vi "Address Bond.vi"(6 "Match Offset":cluster{"X":sgl, "Y":sgl}={"X"=-2.0, "Y"=198.0}, 8 "Minimum Match Score":sgl=60.0, 9 "controller in":refnum<k24>, 10 "Template":path, 11 "T/B/L/R":i32) -> (0 "error out":errorcluster, 1 "Number of Matches (Pattern Matching 1)":i32, 3 "Match(es) Found":bool)   [LabVIEW 2011]
uses:
  C:/Users/Admin/Desktop/Gantry Code Transfer/source/Code Transfer/Aerotech.A3200.dll
  Aerotech.A3200.dll
  <vilib>/vision/driver/NI_Vision_Acquisition_Software.lvlib
  <vilib>/vision/NI_Vision_Development_Module.lvlib
panel:
  in  "Scale Factor":sgl=0.000429
  out "y rel move":dbl
  out "x rel move":dbl
  out "y":sgl
  out "x":sgl
  out "Image Out":T1(plugin-control)
  out "Calibrated Matches (Pattern Matching 1)":T2(array[cluster]) {"Bounding Box"."y" format="%.2f"; "Bounding Box"."x" format="%.2f"; "Position"."y" format="%.2f"; "Position"."x" format="%.2f"; "Score" format="%.2f"; "Scale" format="%.2f"; "Angle" format="%.2f"}
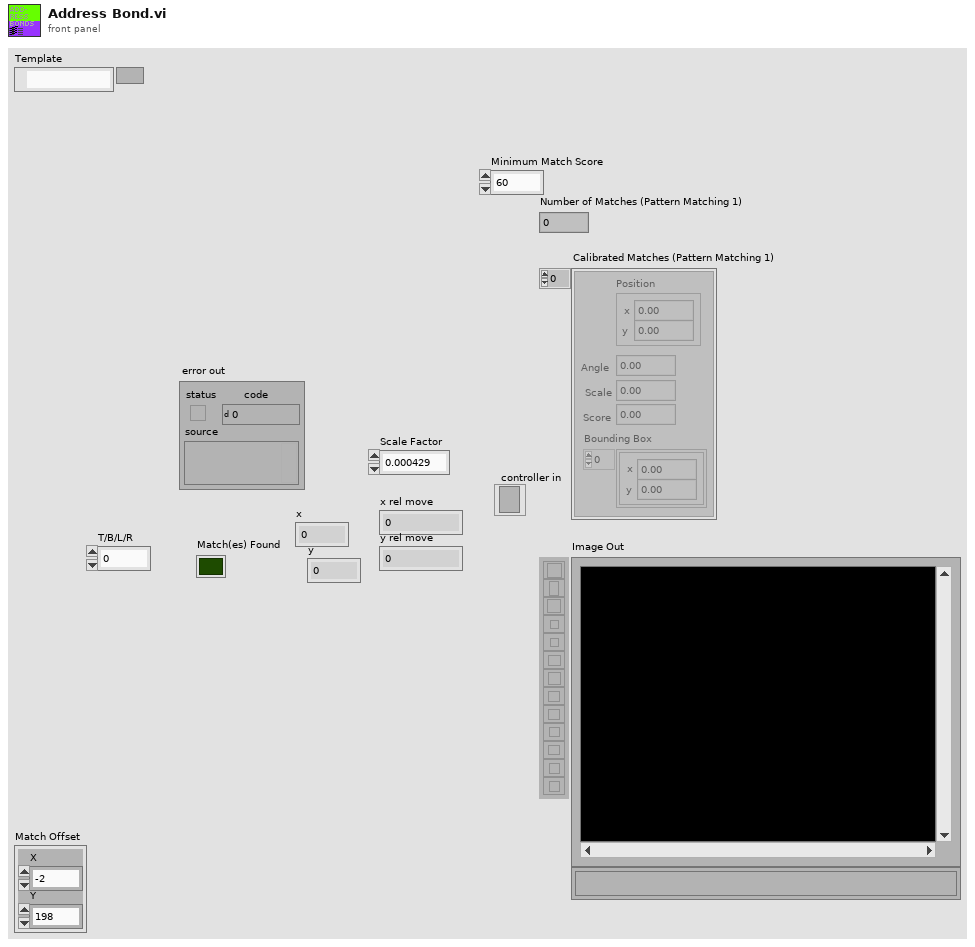
[diagram p1: front panel]
types:
  T1 = typedef "IMAQ Image.ctl" = refnum<image>
  T2 = cluster{"Position":cluster{"x":sgl, "y":sgl}, "Angle":sgl, "Scale":sgl, "Score":sgl, "Bounding Box":cluster{"x":sgl, "y":sgl}[]}[]
  T3 = cluster{"Global Rectangle":i32[], "Contours":cluster{"ID":enum32{"External", "Internal"}, "Type":u32, "Coordinates":i32[]}[]}
  T4 = typedef "IMAQdx.ctl" = refnum<k21>
  T5 = cluster{"Match Mode":u16, "Subpixel Accuracy":bool, "Rotation Angle Ranges (degrees)":cluster{sgl, sgl}[]}
  T6 = cluster{"Global Rectangle":i32[], "Number of Matches Requested":i32, "Minimum Match Score":sgl}
  T7 = cluster{"Position":cluster{"x":sgl, "y":sgl}, "Angle":sgl, "Scale":sgl, "Score":sgl, "Bounding Box":cluster{"x":sgl, "y":sgl}[]}
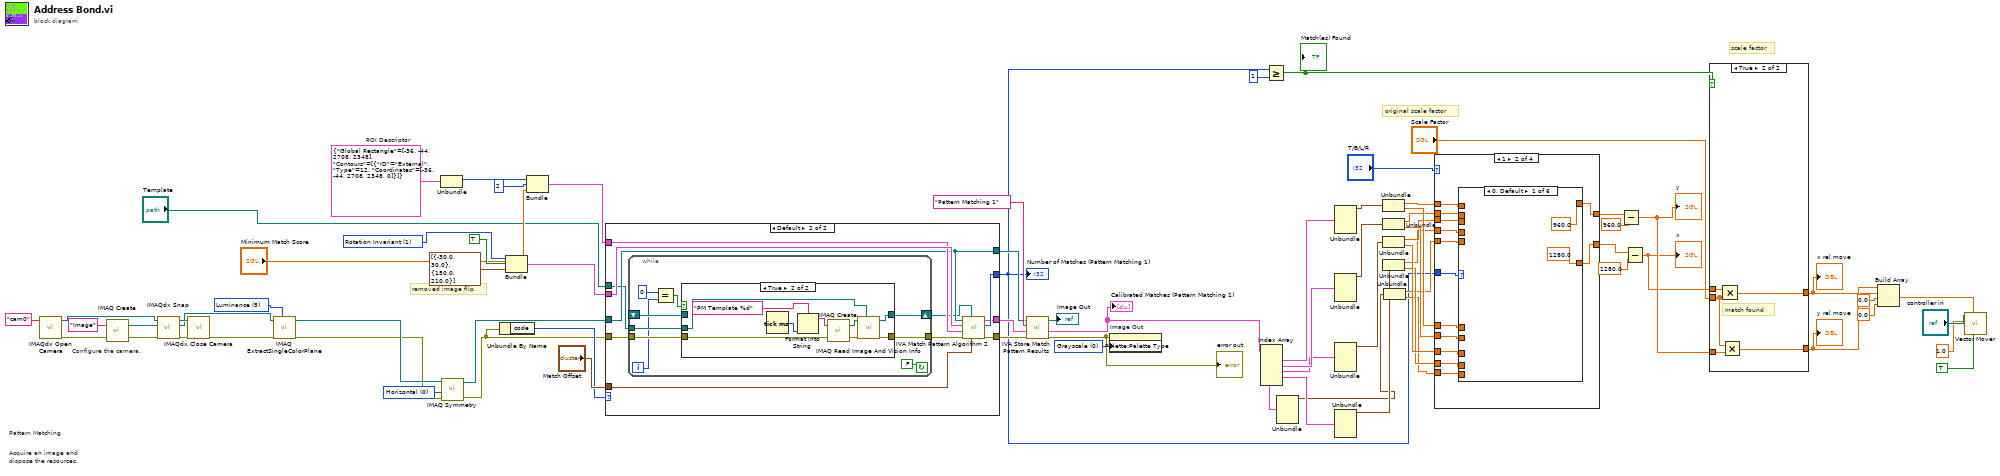
[diagram p0: block diagram]
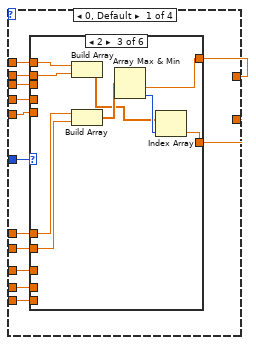
[diagram p2: hidden frame]
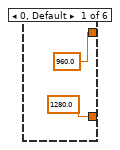
[diagram p3: hidden frame]
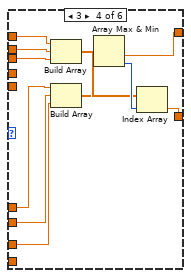
[diagram p5: hidden frame]
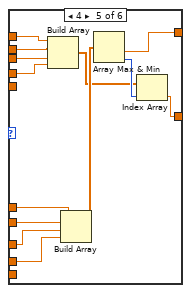
[diagram p6: hidden frame]
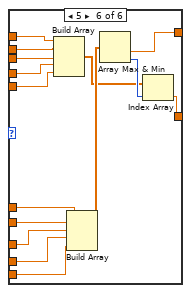
[diagram p7: hidden frame]
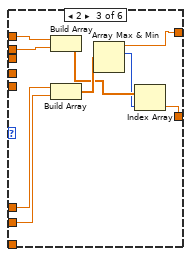
[diagram p9: hidden frame]
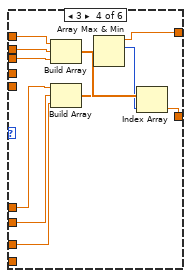
[diagram p10: hidden frame]
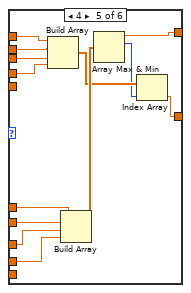
[diagram p11: hidden frame]
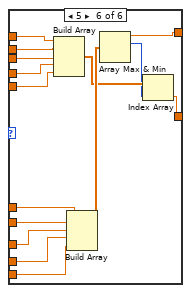
[diagram p12: hidden frame]
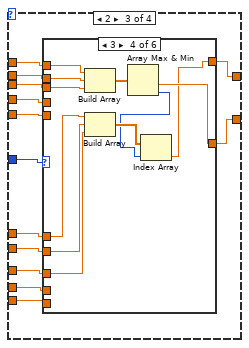
[diagram p13: hidden frame]
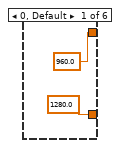
[diagram p14: hidden frame]
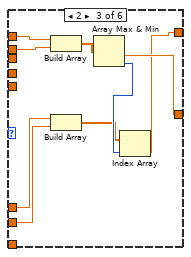
[diagram p16: hidden frame]
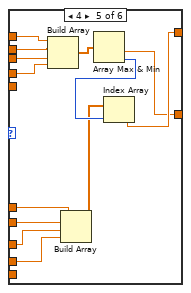
[diagram p17: hidden frame]
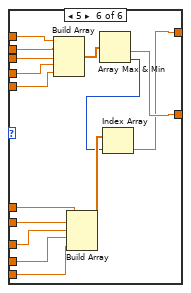
[diagram p18: hidden frame]
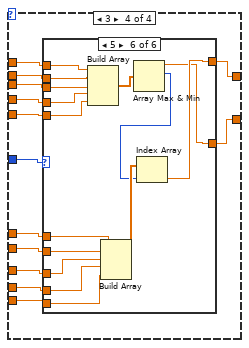
[diagram p19: hidden frame]
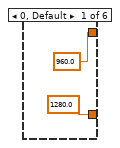
[diagram p20: hidden frame]
diagram:
  w5 = u32 0 items=["Horizontal", "Vertical", "Central", "1st Diagonal", "2nd Diagonal"] ("Type of Symmetry")
  w48 = u32 0 items=["Grayscale", "Binary", "Gradient", "Rainbow", "Temperature", "User Defined"] ("Palette")
  w64 = u16 1 items=["Shift Invariant", "Rotation Invariant"] ("Match Mode")
  w54 = T3 {"Global Rectangle"=[-36, -44, 2708, 2348], "Contours"=[{"ID"=enum."External", "Type"=12, "Coordinates"=[-36, -44, 2708, 2348, 0]}]}  # ROI Descriptor
  w66 = 5 items=["Red", "Green", "Blue", "Hue", "Saturation", "Luminance", "Value", "Intensity"] ("Color Plane")
  # "removed image flip"
  # "original scale factor"
  # "scale factor"
  # "Pattern Matching"
  # "Acquire an image and\ndispose the resources."
  # "Configure the camera."
  n1 = call <vilib>:"IMAQdx Open Camera.vi"("Session In"="cam0" ("Interface Name")) -> ("error out"=w73:errorcluster, "Session Out"=w67:T4)  [unwired: 9 in]
  n2 = call "IMAQ Create"("Image Name"="Image", "error in (no error)"=w73) -> ("New Image"=w69:T1, "error out"=w68:errorcluster)  [unwired: 3 in]
  n3 = call <vilib>:"IMAQdx Snap.vi"("error in"=w68, "Image In"=w69, "Session In"=w67) -> ("error out"=w71:errorcluster, "Image Out"=w65:T1, "Session Out"=w72:T4)  [unwired: 6 in]
  n4 = call <vilib>:"IMAQdx Close Camera.vi"("error in"=w71, "Session In"=w72) -> ("error out"=w70:errorcluster)  [unwired: 9 in]
  n5 = call "IMAQ ExtractSingleColorPlane"("Color Plane"=w66, "error in (no error)"=w70, "Image Src"=w65) -> ("error out"=w3:errorcluster, "Image Dst Out"=w4:T1)  [unwired: 7 in]
  n6 = Unbundle(w54) -> ("Global Rectangle"=w53:i32[])  [unwired: 1 out]
  n7 = call "IMAQ Symmetry"("error in (no error)"=w3, "Type of Symmetry"=w5, "Image Src"=w4) -> ("error out"=w2:errorcluster, "Image Dst Out"=w1:T1)  [unwired: 2 in]
  n8 = Unbundle By Name(w2) -> ("code"=w50:i32)
  n9 = Bundle("Match Mode"=w64, "Subpixel Accuracy"=TRUE, "Rotation Angle Ranges (degrees)"=cluster{sgl, sgl}[] [{-30.0, 30.0}, {150.0, 210.0}]) -> (w61:T5)  [unwired: 1 in]
  n10 = Bundle("Global Rectangle"=w53, "Number of Matches Requested"=2, "Minimum Match Score"="Minimum Match Score") -> (w58:T6)  [unwired: 1 in]
  n11 = case shown="Default" w50 {
    tunnel: "Template" -> [_ w80]
    tunnel: w2 -> [_ w79]
    tunnel: [_ w87] -> w7
    tunnel: w61 -> [_ w86]
    tunnel: w58 -> [_ w85]
    tunnel: "Match Offset" -> [_ w84]
    tunnel: w1 -> [w76 w81]
    tunnel: [_ w83] -> w55
    tunnel: [_ w82] -> w52
    tunnel: [w76 w81] -> w51
    frame -1074396199, -1074396198 {
      # "Discard\nCoordinate\nSystem Error"
    }
    frame Default {
      n12 = while {
        shift-right: [w96] -> w77
        shift-left: _ -> [w95]
        tunnel: [w93] -> w78
        tunnel: w79 -> [w92]
        tunnel: w80 -> [w91]
        i -> [w90]
        stop <- FALSE continue-if-true
        n13 = Equal?(x=0, y=w90) -> (x = y?=w88:bool)
        n14 = case shown="True" w88 {
          tunnel: [w98 w104] -> w96
          tunnel: w95 -> [w98 _]
          tunnel: [w97 w101] -> w93
          tunnel: w92 -> [w97 w100]
          tunnel: w91 -> [_ w99]
          frame False {
          }
          frame True {
            n15 = Tick Count (ms)() -> (millisecond timer value=w107:u32)
            n16 = Format Into String(format string="PM Template %d" ("Image Name"), w107) -> (resulting string=w106:string)  [unwired: 2 in, 1 out]
            n17 = call "IMAQ Create"("Image Name"=w106, "error in (no error)"=w100) -> ("New Image"=w103:T1, "error out"=w102:errorcluster)  [unwired: 3 in]
            n18 = call "IMAQ Read Image And Vision Info"("File Path"=w99, "error in (no error)"=w102, "Image"=w103) -> ("error out"=w101:errorcluster, "Image Out"=w104:T1)  [unwired: 6 in, 1 out]
          }
        }
      }
      n19 = call <vilib>:"IVA Match Pattern Algorithm 2.vi"("Match Offset"=w84, "Image Template"=w77, "error in (no error)"=w78, "Match Parameters"=w85, "Setup Match Parameters"=w86, "Image"=w81) -> ("error out"=w83:errorcluster, "Number of Matches"=w87:i32, "Matches"=w82:T2)  [unwired: 3 in]
    }
  }
  "Number of Matches (Pattern Matching 1)" <- w7
  n20 = call <vilib>:"IVA Store Match Pattern Results.vi"("error in (no error)"=w55, "Matches"=w52, "Step Name"="Pattern Matching 1", "Image in"=w51) -> ("error out"=w8:errorcluster, "Calibrated Matches"=w9:T2, "Image dup"=→"Image Out":T1)  [unwired: 5 in]
  "Calibrated Matches (Pattern Matching 1)" <- w9
  "error out" <- w8
  n21 = property on="Image Out" class="ImageControl"(error in=w8, "Palette:Palette Type"=w48) -> ()  [unwired: 1 in, 2 out]
  n22 = Index Array(array=w9) -> (element #1=w44:T7, element #2=w43:T7, element #3=w42:T7, element #4=w41:T7, element #5=w21:T7)  [unwired: 5 in]
  n23 = Greater Or Equal?(x=w7, y=1) -> (x >= y?=w34:bool)
  "Match(es) Found" <- w34
  n24 = Unbundle(w21) -> ("Position"=w20:cluster{"x":sgl, "y":sgl})  [unwired: 4 out]
  n25 = Unbundle(w44) -> ("Position"=w37:cluster{"x":sgl, "y":sgl})  [unwired: 4 out]
  n26 = Unbundle(w43) -> ("Position"=w38:cluster{"x":sgl, "y":sgl})  [unwired: 4 out]
  n27 = Unbundle(w42) -> ("Position"=w39:cluster{"x":sgl, "y":sgl})  [unwired: 4 out]
  n28 = Unbundle(w41) -> ("Position"=w40:cluster{"x":sgl, "y":sgl})  [unwired: 4 out]
  n29 = Unbundle(w37) -> ("x"=w31:sgl, "y"=w30:sgl)
  n30 = Unbundle(w38) -> ("x"=w29:sgl, "y"=w28:sgl)
  n31 = Unbundle(w39) -> ("x"=w26:sgl, "y"=w25:sgl)
  n32 = Unbundle(w40) -> ("x"=w22:sgl, "y"=w24:sgl)
  n33 = Unbundle(w20) -> ("x"=w19:sgl, "y"=w18:sgl)
  n34 = case shown="1" "T/B/L/R" {
    tunnel: w31 -> [w120 w185 w250 w315]
    tunnel: w30 -> [w119 w180 w245 w310]
    tunnel: w29 -> [w118 w184 w249 w314]
    tunnel: w28 -> [w117 w179 w244 w309]
    tunnel: [w116 w173 w238 w303] -> w27
    tunnel: w26 -> [w115 w183 w248 w313]
    tunnel: w25 -> [w114 w178 w243 w308]
    tunnel: w24 -> [w113 w177 w242 w307]
    tunnel: [w112 w174 w239 w304] -> w23
    tunnel: w22 -> [w111 w182 w247 w312]
    tunnel: w19 -> [w110 w181 w246 w311]
    tunnel: w18 -> [w109 w176 w241 w306]
    tunnel: w7 -> [w108 w175 w240 w305]
    frame 0, Default {
      n35 = case shown="2" w108 {
        tunnel: w120 -> [_ w123 w133 w141 w154 w169]
        tunnel: w119 -> [_ w124 w131 w138 w150 w165]
        tunnel: [sgl 960.0 ("y") w124 w128 w143 w156 w171] -> w116
        tunnel: w118 -> [_ _ w132 w140 w153 w168]
        tunnel: w117 -> [_ _ w130 w137 w149 w164]
        tunnel: w115 -> [_ _ _ w139 w152 w167]
        tunnel: w114 -> [_ _ _ w136 w148 w163]
        tunnel: w113 -> [_ _ _ _ w147 w162]
        tunnel: [sgl 1280.0 ("x") w123 w125 w142 w155 w170] -> w112
        tunnel: w111 -> [_ _ _ _ w151 w166]
        tunnel: w110 -> [_ _ _ _ _ w159]
        tunnel: w109 -> [_ _ _ _ _ w158]
        frame 0, Default {
        }
        frame 1 {
        }
        frame 2 {
          n36 = Build Array(w133, w132) -> (w126:sgl[])
          n37 = Build Array(w131, w130) -> (w127:sgl[])
          n38 = Array Max & Min(array=w127) -> (min value=w128:sgl, min index (indices)=w129:i32)  [unwired: 2 out]
          n39 = Index Array(array=w126, index=w129) -> (element=w125:sgl)
        }
        frame 3 {
          n40 = Build Array(w141, w140, w139) -> (w135:sgl[])
          n41 = Build Array(w138, w137, w136) -> (w134:sgl[])
          n42 = Array Max & Min(array=w134) -> (min value=w143:sgl, min index (indices)=w144:i32)  [unwired: 2 out]
          n43 = Index Array(array=w135, index=w144) -> (element=w142:sgl)
        }
        frame 4 {
          n44 = Build Array(w154, w153, w152, w151) -> (w145:sgl[])
          n45 = Build Array(w150, w149, w148, w147) -> (w146:sgl[])
          n46 = Array Max & Min(array=w146) -> (min value=w156:sgl, min index (indices)=w157:i32)  [unwired: 2 out]
          n47 = Index Array(array=w145, index=w157) -> (element=w155:sgl)
        }
        frame 5 {
          n48 = Build Array(w169, w168, w167, w166, w159) -> (w160:sgl[])
          n49 = Build Array(w165, w164, w163, w162, w158) -> (w161:sgl[])
          n50 = Array Max & Min(array=w161) -> (min value=w171:sgl, min index (indices)=w172:i32)  [unwired: 2 out]
          n51 = Index Array(array=w160, index=w172) -> (element=w170:sgl)
        }
      }
    }
    frame 1 {
      n52 = case shown="0, Default" w175 {
        tunnel: w185 -> [_ w188 w198 w208 w221 w236]
        tunnel: w180 -> [_ w189 w196 w205 w217 w232]
        tunnel: [sgl 960.0 ("y") w189 w191 w200 w211 w224] -> w173
        tunnel: w184 -> [_ _ w197 w207 w220 w235]
        tunnel: w179 -> [_ _ w195 w204 w216 w231]
        tunnel: w183 -> [_ _ _ w206 w219 w234]
        tunnel: w178 -> [_ _ _ w203 w215 w230]
        tunnel: w177 -> [_ _ _ _ w214 w229]
        tunnel: [sgl 1280.0 ("x") w188 w192 w209 w222 w237] -> w174
        tunnel: w182 -> [_ _ _ _ w218 w233]
        tunnel: w181 -> [_ _ _ _ _ w226]
        tunnel: w176 -> [_ _ _ _ _ w225]
        frame 0, Default {
        }
        frame 1 {
        }
        frame 2 {
          n53 = Build Array(w198, w197) -> (w193:sgl[])
          n54 = Build Array(w196, w195) -> (w194:sgl[])
          n55 = Array Max & Min(array=w194) -> (max value=w191:sgl, max index (indices)=w190:i32)  [unwired: 2 out]
          n56 = Index Array(array=w193, index=w190) -> (element=w192:sgl)
        }
        frame 3 {
          n57 = Build Array(w208, w207, w206) -> (w202:sgl[])
          n58 = Build Array(w205, w204, w203) -> (w201:sgl[])
          n59 = Array Max & Min(array=w201) -> (max value=w200:sgl, max index (indices)=w199:i32)  [unwired: 2 out]
          n60 = Index Array(array=w202, index=w199) -> (element=w209:sgl)
        }
        frame 4 {
          n61 = Build Array(w221, w220, w219, w218) -> (w212:sgl[])
          n62 = Build Array(w217, w216, w215, w214) -> (w213:sgl[])
          n63 = Array Max & Min(array=w213) -> (max value=w211:sgl, max index (indices)=w210:i32)  [unwired: 2 out]
          n64 = Index Array(array=w212, index=w210) -> (element=w222:sgl)
        }
        frame 5 {
          n65 = Build Array(w236, w235, w234, w233, w226) -> (w227:sgl[])
          n66 = Build Array(w232, w231, w230, w229, w225) -> (w228:sgl[])
          n67 = Array Max & Min(array=w228) -> (max value=w224:sgl, max index (indices)=w223:i32)  [unwired: 2 out]
          n68 = Index Array(array=w227, index=w223) -> (element=w237:sgl)
        }
      }
    }
    frame 2 {
      n69 = case shown="3" w240 {
        tunnel: w250 -> [_ w253 w263 w274 w286 w302]
        tunnel: w245 -> [_ w254 w261 w271 w282 w298]
        tunnel: [sgl 960.0 ("y") w254 w255 w264 w276 w288] -> w238
        tunnel: w249 -> [_ _ w262 w273 w285 w301]
        tunnel: w244 -> [_ _ w260 w270 w281 w297]
        tunnel: w248 -> [_ _ _ w272 w284 w300]
        tunnel: w243 -> [_ _ _ w269 w280 w296]
        tunnel: w242 -> [_ _ _ _ w279 w295]
        tunnel: [sgl 1280.0 ("x") w253 w258 w265 w275 w289] -> w239
        tunnel: w247 -> [_ _ _ _ w283 w299]
        tunnel: w246 -> [_ _ _ _ _ w294]
        tunnel: w241 -> [_ _ _ _ _ w293]
        frame 0, Default {
        }
        frame 1 {
        }
        frame 2 {
          n70 = Build Array(w263, w262) -> (w259:sgl[])
          n71 = Build Array(w261, w260) -> (w256:sgl[])
          n72 = Array Max & Min(array=w259) -> (min value=w258:sgl, min index (indices)=w257:i32)  [unwired: 2 out]
          n73 = Index Array(array=w256, index=w257) -> (element=w255:sgl)
        }
        frame 3 {
          n74 = Build Array(w274, w273, w272) -> (w268:sgl[])
          n75 = Build Array(w271, w270, w269) -> (w267:sgl[])
          n76 = Array Max & Min(array=w268) -> (min value=w265:sgl, min index (indices)=w266:i32)  [unwired: 2 out]
          n77 = Index Array(array=w267, index=w266) -> (element=w264:sgl)
        }
        frame 4 {
          n78 = Build Array(w286, w285, w284, w283) -> (w277:sgl[])
          n79 = Build Array(w282, w281, w280, w279) -> (w278:sgl[])
          n80 = Array Max & Min(array=w277) -> (min value=w275:sgl, min index (indices)=w287:i32)  [unwired: 2 out]
          n81 = Index Array(array=w278, index=w287) -> (element=w276:sgl)
        }
        frame 5 {
          n82 = Build Array(w302, w301, w300, w299, w294) -> (w290:sgl[])
          n83 = Build Array(w298, w297, w296, w295, w293) -> (w292:sgl[])
          n84 = Array Max & Min(array=w290) -> (min value=w289:sgl, min index (indices)=w291:i32)  [unwired: 2 out]
          n85 = Index Array(array=w292, index=w291) -> (element=w288:sgl)
        }
      }
    }
    frame 3 {
      n86 = case shown="5" w305 {
        tunnel: w315 -> [_ w318 w328 w339 w352 w367]
        tunnel: w310 -> [_ w319 w326 w336 w348 w363]
        tunnel: [sgl 960.0 ("y") w319 w322 w331 w342 w355] -> w303
        tunnel: w314 -> [_ _ w327 w338 w351 w366]
        tunnel: w309 -> [_ _ w325 w335 w347 w362]
        tunnel: w313 -> [_ _ _ w337 w350 w365]
        tunnel: w308 -> [_ _ _ w334 w346 w361]
        tunnel: w307 -> [_ _ _ _ w345 w360]
        tunnel: [sgl 1280.0 ("x") w318 w321 w330 w341 w354] -> w304
        tunnel: w312 -> [_ _ _ _ w349 w364]
        tunnel: w311 -> [_ _ _ _ _ w359]
        tunnel: w306 -> [_ _ _ _ _ w358]
        frame 0, Default {
        }
        frame 1 {
        }
        frame 2 {
          n87 = Build Array(w328, w327) -> (w324:sgl[])
          n88 = Build Array(w326, w325) -> (w323:sgl[])
          n89 = Array Max & Min(array=w324) -> (max value=w321:sgl, max index (indices)=w320:i32)  [unwired: 2 out]
          n90 = Index Array(array=w323, index=w320) -> (element=w322:sgl)
        }
        frame 3 {
          n91 = Build Array(w339, w338, w337) -> (w333:sgl[])
          n92 = Build Array(w336, w335, w334) -> (w332:sgl[])
          n93 = Array Max & Min(array=w333) -> (max value=w330:sgl, max index (indices)=w329:i32)  [unwired: 2 out]
          n94 = Index Array(array=w332, index=w329) -> (element=w331:sgl)
        }
        frame 4 {
          n95 = Build Array(w352, w351, w350, w349) -> (w343:sgl[])
          n96 = Build Array(w348, w347, w346, w345) -> (w344:sgl[])
          n97 = Array Max & Min(array=w343) -> (max value=w341:sgl, max index (indices)=w340:i32)  [unwired: 2 out]
          n98 = Index Array(array=w344, index=w340) -> (element=w342:sgl)
        }
        frame 5 {
          n99 = Build Array(w367, w366, w365, w364, w359) -> (w356:sgl[])
          n100 = Build Array(w363, w362, w361, w360, w358) -> (w357:sgl[])
          n101 = Array Max & Min(array=w356) -> (max value=w354:sgl, max index (indices)=w353:i32)  [unwired: 2 out]
          n102 = Index Array(array=w357, index=w353) -> (element=w355:sgl)
        }
      }
    }
  }
  n103 = Subtract(x=w27, y=sgl 960.0) -> (x-y=w47:sgl)
  "y" <- w47
  n104 = Subtract(x=w23, y=sgl 1280.0) -> (x-y=w46:sgl)
  "x" <- w46
  n105 = case shown="True" w34 {
    tunnel: w47 -> [_ w373]
    tunnel: w46 -> [_ w372]
    tunnel: [w368 w371] -> w32
    tunnel: [w368 w370] -> w33
    tunnel: "Scale Factor" -> [_ w369]
    frame False {
      w368 = sgl 0.0
      # "no match found"
    }
    frame True {
      # "match found"
      n106 = Multiply(x=w372, y=w369) -> (x*y=w371:sgl)
      n107 = Multiply(x=w369, y=w373) -> (x*y=w370:sgl)
    }
  }
  "x rel move" <- w32
  "y rel move" <- w33
  n108 = Build Array(w33, w32, 0.0 ("element"), 0.0 ("element")) -> (w10:dbl[])
  n109 = call "Vector Mover.vi"("Absolute/Relative (F/T)"=TRUE, "Movement Vector"=w10, "Vector Speed"=1.0, "controller in"="controller in") -> ()  [unwired: 2 in, 4 out]
